vi "DBL Aray to JSON.vi"(7 "enable LabVIEW extensions?":bool, 11 "DBL Array":dbl[](array[numeric])) -> (3 "<JSON>Array":string)   [LabVIEW 2020, in "JSONtext.lvlib"]
uses:
  <vilib>/JDP Science/JSONtext/JSONtext.lvlib
  <vilib>/JDP Science/JSONtext/support/Remove trailing zeros.vi
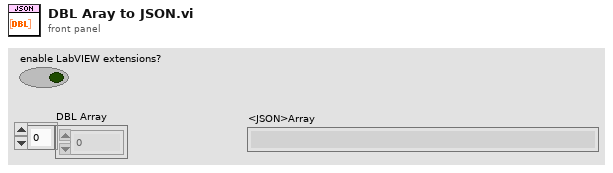
[diagram p1: front panel]
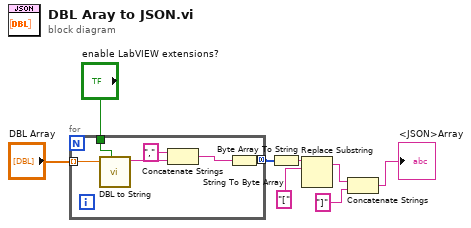
[diagram p0: block diagram]
diagram:
  n1 = for {
    tunnel: "DBL Array" -> [w14] mode=indexing
    tunnel: "enable LabVIEW extensions?" -> [w13]
    tunnel: [w11] -> w6 mode=concatenating
    n2 = call <vilib>:"DBL to String.vi"("enable LabVIEW extensions?"=w13, "DBL"=w14) -> ("DBL string"=w12:string)  [unwired: 9 in]
    n3 = Concatenate Strings("," ("string"), w12) -> (w10:string)
    n4 = String To Byte Array(string=w10) -> (unsigned byte array=w11:u8[])
  }
  n5 = Byte Array To String(unsigned byte array=w6) -> (string=w7:string)
  n6 = Replace Substring(4:"[" ("substring (\"\")"), 5:w7) -> (1:w3:string)  [unwired: 2 in, 1 out]
  n7 = Concatenate Strings(w3, "]" ("string")) -> (→"<JSON>Array":string)
